vi "DAQ_active_to_global_channels.vi"(10 "Active Channels":tag[](array[tag])) -> (2 "Global Channels":refnum<k21>)   [LabVIEW 2016]
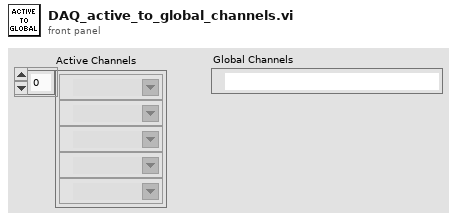
[diagram p1: front panel]
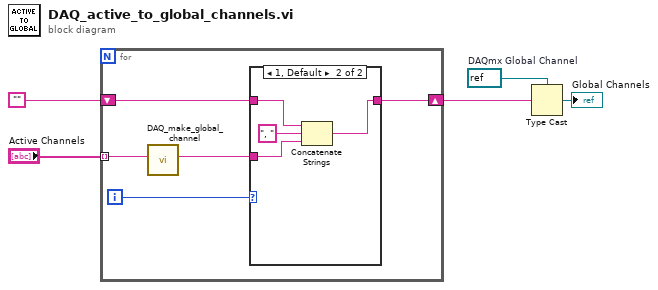
[diagram p0: block diagram]
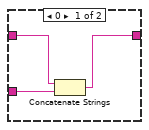
[diagram p2: hidden frame]
diagram:
  w2 = refnum<k21> refnum  # DAQmx Global Channel
  n1 = for {
    tunnel: "Active Channels" -> [w10] mode=indexing
    shift-right: [w6] -> w3
    shift-left: "" -> [w9]
    i -> [w7]
    n2 = call "DAQ_make_global_channel.vi"("DAQmx Physical Channel"=w10) -> ("concatenated string"=w8:string)  [unwired: 10 in]
    n3 = case shown="1, Default" w7 {
      tunnel: w9 -> [w13 w17]
      tunnel: w8 -> [w12 w15]
      tunnel: [w11 w14] -> w6
      frame 0 {
        n4 = Concatenate Strings(w13, w12) -> (w11:string)
      }
      frame 1, Default {
        n5 = Concatenate Strings(w17, ", " ("string"), w15) -> (w14:string)
      }
    }
  }
  n6 = Type Cast(type=w2, x=w3) -> (*(type *) &x=→"Global Channels":refnum<k21>)
